vi "move shoulder from initializatiion.vi"   [LabVIEW 2015]
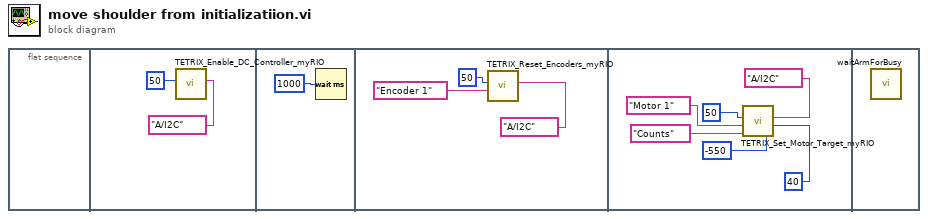
[diagram p0: block diagram]
diagram:
  n1 = flat-sequence {
    frame #0 {
    }
    frame #1 {
      n2 = call <vilib>:"TETRIX_Enable_DC_Controller_myRIO.vi"("myRIO MXP Port A/B"=tag "A/I2C", "Controller ID#  (I2C Address)"=u8 50) -> ()  [unwired: 5 in, 1 out]
    }
    frame #2 {
      n3 = Wait (ms)(milliseconds to wait=u32 1000) -> ()  [unwired: 1 out]
    }
    frame #3 {
      n4 = call <vilib>:"TETRIX_Reset_Encoders_myRIO.vi"("myRIO MXP Port A/B"=tag "A/I2C", "Select Encoder"="Encoder 1", "Controller ID#  (I2C Address)"=u8 50) -> ()  [unwired: 4 in, 1 out]
    }
    frame #4 {
      n5 = call <vilib>:"TETRIX_Set_Motor_Target_myRIO.vi"("Motor Encoder Target"=-550, "Constant Speed (Degrees per Second)"=i16 40, "myRIO MXP Port A/B"=tag "A/I2C", "Encoder Units"="Counts", "Select Channel"="Motor 1", "Controller ID#  (I2C Address)"=u8 50) -> ()  [unwired: 1 in, 1 out]
    }
    frame #5 {
      n6 = call "waitArmForBusy.vi"() -> ()  [unwired: 12 in]
    }
  }
